vi "Configure Channel Core.vi"(0 "CS++Scope":refnum<class "CS++Scope.lvclass">, 1 "channel enabled (True)":bool=TRUE, 2 "channel name (\"CHANNEL1\")":string="CHANNEL1", 3 "probe attenuation (1:1.0)":dbl=1.0 format="%.3f", 4 "vertical offset (0.0 V)":dbl[unit] format="%.3f", 5 "error in (no error)":errorcluster, 6 "vertical coupling (DC)":i32(ring)=1 items=["AC", "DC", "GND"], 8 "vertical range (10.0 V)":dbl[unit]=10.0 format="%.3f") -> (14 "CS++Scope out":refnum<class "CS++Scope.lvclass">, 19 "error out":errorcluster)   [LabVIEW 2013, in "CS++Scope.lvlib" / "CS++Scope.lvclass"]
doc: "This VI configures the most commonly configured properties of the oscilloscope channel sub-system. These properties are the range, offset, coupling, probe attenuation, and whether the channel is enabled."
uses:
  CS++Scope.lvclass
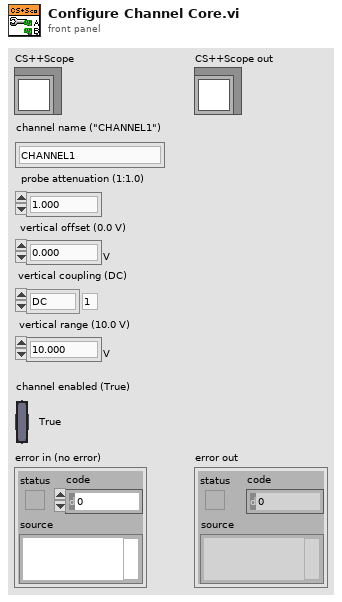
[diagram p1: front panel]
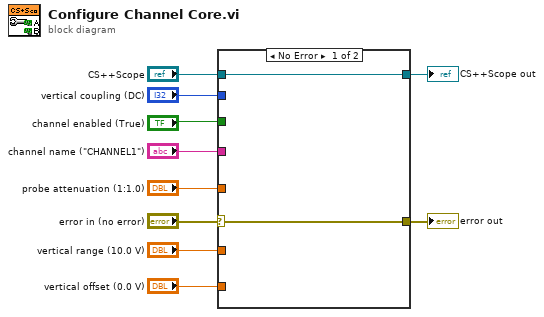
[diagram p0: block diagram]
diagram:
  n1 = case shown="No Error" "error in (no error)" {
    selector: "error in (no error)" -> [w11 w14]
    tunnel: [w11 w14] -> w9
    tunnel: [w12 w13] -> w2
    tunnel: "CS++Scope" -> [w12 w13]
    tunnel: "channel name (\"CHANNEL1\")" -> [_ _]
    tunnel: "probe attenuation (1:1.0)" -> [_ _]
    tunnel: "vertical range (10.0 V)" -> [_ _]
    tunnel: "vertical offset (0.0 V)" -> [_ _]
    tunnel: "channel enabled (True)" -> [_ _]
    tunnel: "vertical coupling (DC)" -> [_ _]
    frame No Error {
    }
    frame Error {
    }
  }
  "error out" <- w9
  "CS++Scope out" <- w2
